vi "test_isRunningShouldWorkEvenIfTaskStoppedPrematurely.vi"(11 "Test Case In":refnum<class "TaskControllerTests.lvclass">) -> (0 "error out":errorcluster, 3 "Test Case Out":refnum<class "TaskControllerTests.lvclass">)   [LabVIEW 2023, in "TaskControllerTests.lvclass"]
uses:
  TaskControllerTests.lvclass
  TaskControllerTests.lvclass/TaskControllerTests.ctl
  TaskMock/TaskMock.lvclass
  <vilib>/Astemes/LUnit/Test Case.lvclass
  source/TaskController/TaskController.lvclass
  C:/projects/TLC_Daemon/tests/TaskMock/TaskMock.lvclass
  C:/projects/TLC_Daemon/source/ITask/ITask.lvclass
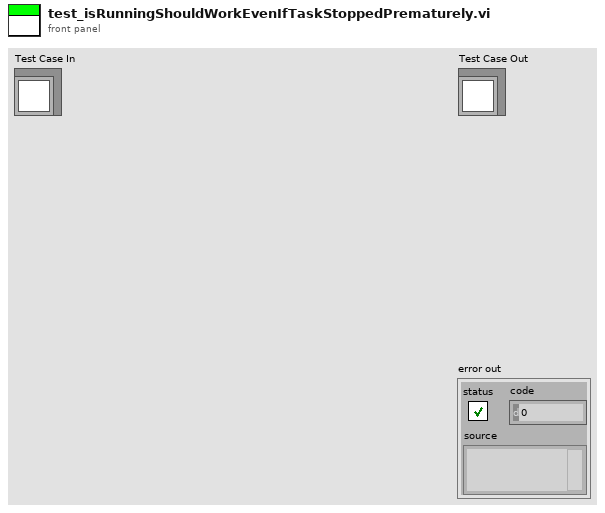
[diagram p1: front panel]
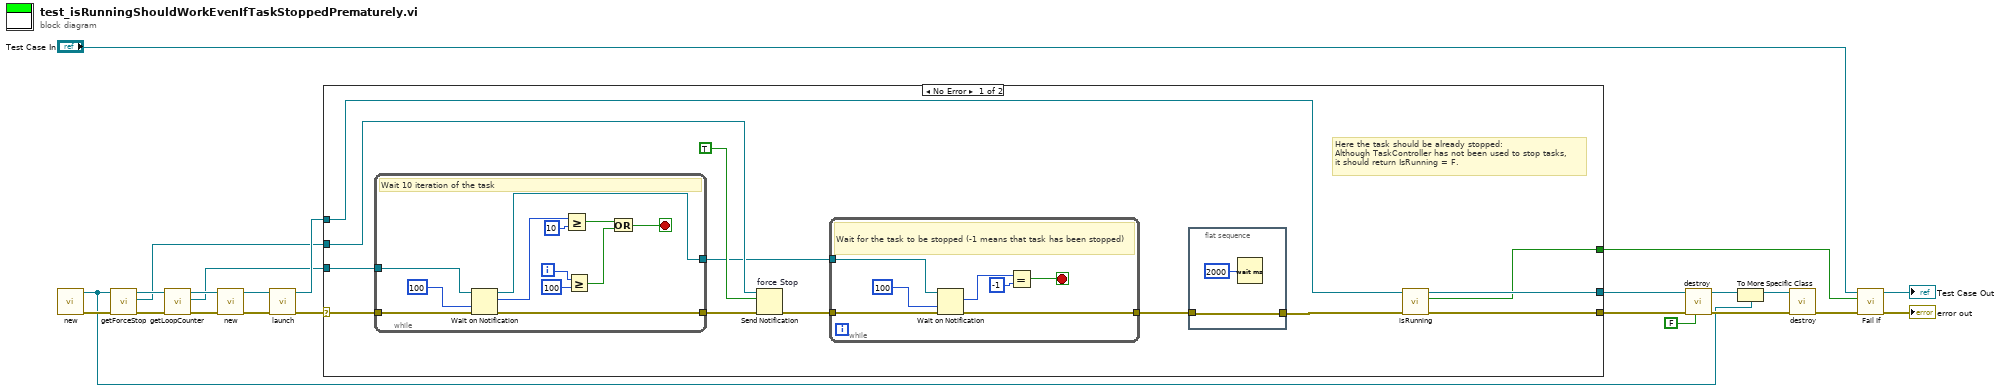
[diagram p0: block diagram]
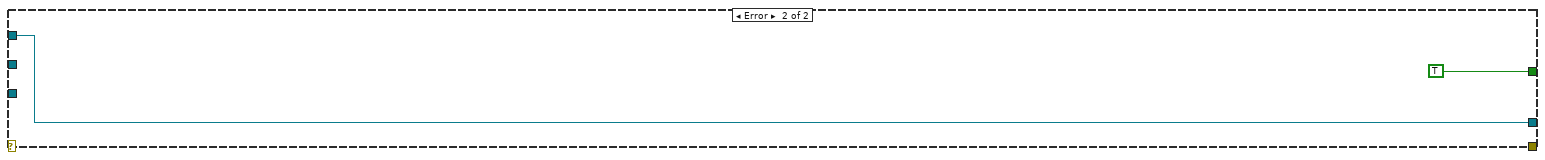
[diagram p2: hidden frame]
diagram:
  n1 = call "new.vi"() -> ("error out"=w9:errorcluster, "TaskMock out"=w4:refnum<class "TaskMock.lvclass">)  [unwired: 10 in]
  n2 = call "getForceStop.vi"("error in (no error)"=w9, "TaskMock in"=w4) -> ("error out"=w6:errorcluster, "forceStop"=w3:refnum<notifier>, "TaskMock out"=w5:refnum<class "TaskMock.lvclass">)  [unwired: 7 in]
  n3 = call "getLoopCounter.vi"("error in (no error)"=w6, "TaskMock in"=w5) -> ("error out"=w8:errorcluster, "loopCounter"=w15:refnum<notifier>, "TaskMock out"=w16:refnum<class "TaskMock.lvclass">)  [unwired: 7 in]
  n4 = call "new.vi"("error in (no error)"=w8, "task"=w16) -> ("error out"=w19:errorcluster, "TaskController out"=w20:refnum<class "TaskController.lvclass">)  [unwired: 8 in]
  n5 = call "launch.vi"("error in (no error)"=w19, "TaskController in"=w20) -> ("error out"=w17:errorcluster, "TaskController out"=w18:refnum<class "TaskController.lvclass">)  [unwired: 8 in]
  n6 = case shown="No Error" w17 {
    selector: w17 -> [w36 _]
    tunnel: w18 -> [w27 w59]
    tunnel: w15 -> [w35 _]
    tunnel: [w28 w59] -> w14
    tunnel: [w29 _] -> w13
    tunnel: w3 -> [w34 _]
    tunnel: [w26 TRUE ("isRunning")] -> w2
    frame No Error {
      # "Here the task should be already stopped:\nAlthough TaskController has not been used to stop tasks,\nit should return IsRunning = F."
      n7 = while {
        tunnel: w36 -> [w48]
        tunnel: w35 -> [w57]
        tunnel: [w47] -> w32
        tunnel: [w46] -> w30
        i -> [w53]
        stop <- w50 stop-if-true
        # "Wait 10 iteration of the task"
        n8 = Wait on Notification(notifier=w57, timeout in ms (-1)=100, error in (no error)=w48) -> (notifier out=w46:refnum<notifier>, notification=w55:i32, error out=w47:errorcluster)  [unwired: 1 in, 1 out]
        n9 = Greater Or Equal?(x=w55, y=10) -> (x >= y?=w51:bool)
        n10 = Greater Or Equal?(x=w53, y=100) -> (x >= y?=w49:bool)
        n11 = Or(x=w51, y=w49) -> (x .or. y?=w50:bool)
      }
      n12 = Send Notification "force Stop"(notification=TRUE, notifier=w34, error in (no error)=w32) -> (error out=w31:errorcluster)  [unwired: 1 out]
      n13 = while {
        tunnel: w31 -> [w42]
        tunnel: w30 -> [w45]
        tunnel: [w41] -> w25
        stop <- w39 stop-if-true
        # "Wait for the task to be stopped (-1 means that task has been stopped)"
        n14 = Wait on Notification(notifier=w45, timeout in ms (-1)=100, error in (no error)=w42) -> (notification=w43:i32, error out=w41:errorcluster)  [unwired: 1 in, 2 out]
        n15 = Equal?(x=w43, y=-1) -> (x = y?=w39:bool)
      }
      n16 = flat-sequence {
        tunnel: w25 -> [w38]
        tunnel: [w38] -> w24
        frame #0 {
          n17 = Wait (ms)(milliseconds to wait=u32 2000) -> ()  [unwired: 1 out]
        }
      }
      n18 = call "isRunning.vi"("error in (no error)"=w24, "TaskController in"=w27) -> ("error out"=w29:errorcluster, "isRunning"=w26:bool, "TaskController out"=w28:refnum<class "TaskController.lvclass">)  [unwired: 7 in]
    }
    frame Error {
    }
  }
  n19 = call "destroy.vi"("destroyStopMechanism"=FALSE, "error in (no error)"=w13, "TaskController in"=w14) -> ("error out"=w12:errorcluster, "task"=w11:refnum<class "ITask.lvclass">)  [unwired: 7 in]
  n20 = To More Specific Class(target class=w4, reference=w11) -> (specific class reference=w10:refnum<class "TaskMock.lvclass">)  [unwired: 1 in, 1 out]
  n21 = call "destroy.vi"("error in (no error)"=w12, "TaskMock in"=w10) -> ("error out"=w7:errorcluster)  [unwired: 9 in]
  n22 = call <vilib>:"Fail If.vi"("error in (no error)"=w7, "Fail?"=w2, "LUnit Test Case In"="Test Case In") -> ("error out"=→"error out":errorcluster, "LUnit Test Case Out"=→"Test Case Out":refnum<class "TaskControllerTests.lvclass">)  [unwired: 7 in]
